vi "Class - Memory.vi"(7 "Msg Chain":string, 8 "error in (no error)":errorcluster {"code" format="Error %.0f"}, 10 "Classes":refnum<class "Class Documentation.lvclass">[](array[class]), 11 "VIDoc Printer - Confluence In":refnum<class "VIDoc Printer - Confluence.lvclass">) -> (0 "error out":errorcluster {"code" format="Error %.0f"}, 3 "VIDoc Printer - Confluence Out":refnum<class "VIDoc Printer - Confluence.lvclass">)   [LabVIEW 2023, in "VIDoc Printer - Confluence.lvlib" / "VIDoc Printer - Confluence.lvclass"]
uses:
  VIDoc Printer - Confluence.lvclass
  Parsing/Class Documentation/Class Documentation.lvclass
  Confluence Formatting/Types/Format Combo Box.ctl
  Parsing/Class Documentation/Get Total Data Size.vi
  VIDoc Printer - Confluence.lvclass/VIDoc Printer - Confluence.ctl
  Confluence Formatting/Confluence Formatting.lvlib
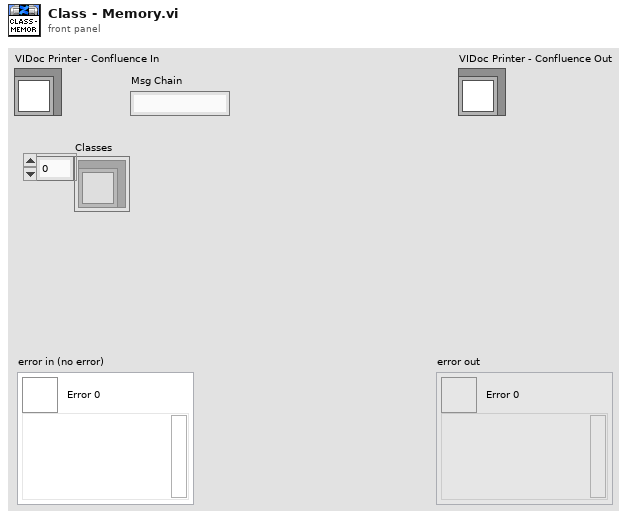
[diagram p1: front panel]
types:
  T1 = typedef "Confluence Formatting.lvlib/Format Combo Box.ctl" = string
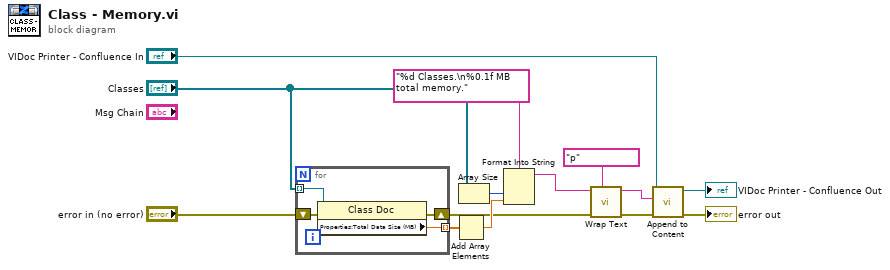
[diagram p0: block diagram]
diagram:
  n1 = for {
    tunnel: "Classes" -> [w17] mode=indexing
    tunnel: [w16] -> w13 mode=indexing
    shift-right: [w15] -> w6
    shift-left: "error in (no error)" -> [w18]
    n2 = property class="Class Doc"(reference=w17, error in=w18) -> (error out=w15:errorcluster, "Properties:Total Data Size (MB)"=w16:dbl)  [unwired: 1 out]
  }
  n3 = Add Array Elements(numeric array=w13) -> (sum=w8:dbl)
  n4 = Array Size(array="Classes") -> (size(s)=w9:i32)
  n5 = Format Into String(format string="%d Classes.\n%0.1f MB total memory.", w9, w8) -> (resulting string=w11:string)  [unwired: 2 in, 1 out]
  n6 = call "Wrap Text.vi"("Formatting"=T1 "p", "Error in"=w6, "String"=w11) -> ("Error out"=w14:errorcluster, "Wrapped String"=w5:string)  [unwired: 7 in]
  n7 = call "Append to Content.vi"("error in (no error)"=w14, "Content"=w5, "VIDoc Printer - Confluence In"="VIDoc Printer - Confluence In") -> ("error out"=→"error out":errorcluster, "VIDoc Printer - Confluence Out"=→"VIDoc Printer - Confluence Out":refnum<class "VIDoc Printer - Confluence.lvclass">)  [unwired: 7 in]
